vi "display color.vi"(6 "Existing fill color":u32 format="%.0x", 7 "Current":dbl format="%.5f", 8 "Field":dbl format="%.5f") -> (0 "Fill Color":u32 format="%.0x", 2 "Current":cluster{dbl, dbl}(slide)={0.0, -0.0065359477124182705} scale=-27.1091940291997..27.1091940291997 scale format="%.1f", 3 "Field":cluster{dbl, dbl}(slide)={0.0, -0.0065359477124182705} scale=-27.1091940291997..27.1091940291997 scale format="%.1f")   [LabVIEW 2019]
panel:
  out "Old current":dbl format="%.5f"
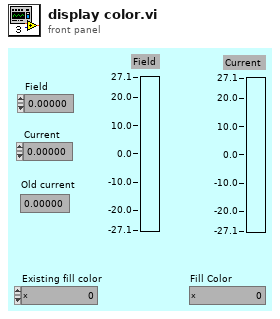
[diagram p1: front panel]
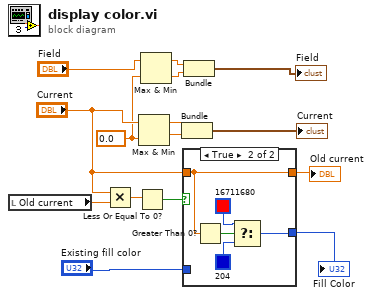
[diagram p0: block diagram]
diagram:
  w2 = 0.0 ("y")
  n1 = local read "Old current"() -> (w12:dbl)
  n2 = Multiply(x="Current", y=w12) -> (x*y=w11:dbl)
  n3 = Less Or Equal To 0?(x=w11) -> (x <= 0?=w8:bool)
  n4 = Max & Min(x="Current", y=w2) -> (max(x,y)=w14:dbl, min(x,y)=w13:dbl)
  n5 = Max & Min(x="Field", y=w2) -> (max(x,y)=w4:dbl, min(x,y)=w3:dbl)
  n6 = Bundle(w14, w13) -> (→"Current":cluster{dbl, dbl})  [unwired: 1 in]
  n7 = case shown="True" w8 {
    tunnel: [w17 w22] -> w9
    tunnel: "Current" -> [w17 w22]
    tunnel: [w16 w18] -> w7
    tunnel: "Existing fill color" -> [w16 _]
    frame False {
    }
    frame True {
      n8 = Greater Than 0?(x=w22) -> (x > 0?=w21:bool)
      n9 = Select(t=u32 16711680, s=w21, f=u32 204) -> (s? t:f=w18:u32)
    }
  }
  "Old current" <- w9
  "Fill Color" <- w7
  n10 = Bundle(w4, w3) -> (→"Field":cluster{dbl, dbl})  [unwired: 1 in]
